vi "SeleccionarEntrada.vi"(6 "error in (no error)":errorcluster, 9 "DAQ in":refnum<class "DAQ.lvclass">) -> (0 "error out":errorcluster, 3 "DAQ out":refnum<class "DAQ.lvclass">)   [LabVIEW 2019, in "DAQ.lvclass"]
uses:
  DAQ.lvclass
  <resource>/objmgr/daqmx.rc
  <vilib>/DAQmx/create/channels.llb/DAQmx Create Channel (AI-Voltage-Basic).vi
  <vilib>/DAQmx/configure/timing.llb/DAQmx Timing (Sample Clock).vi
panel:
  out "SampClk.Rate":dbl
  in  "Number of Samples":i32=100
  in  "Sample Rate":dbl=1000.0
  in  "Sample Clock Source":tag="OnboardClock"
  in  "Terminal Configuration":i32(ring)=-1 items=["default"=-1, "RSE"=10083, "NRSE"=10078, "Differential"=10106, "Pseudodifferential"=12529]
  in  "Max Voltage":dbl=5.0
  in  "Min Voltage":dbl=-5.0
  in  "Physical Channel":tag="Dev1/ai0"
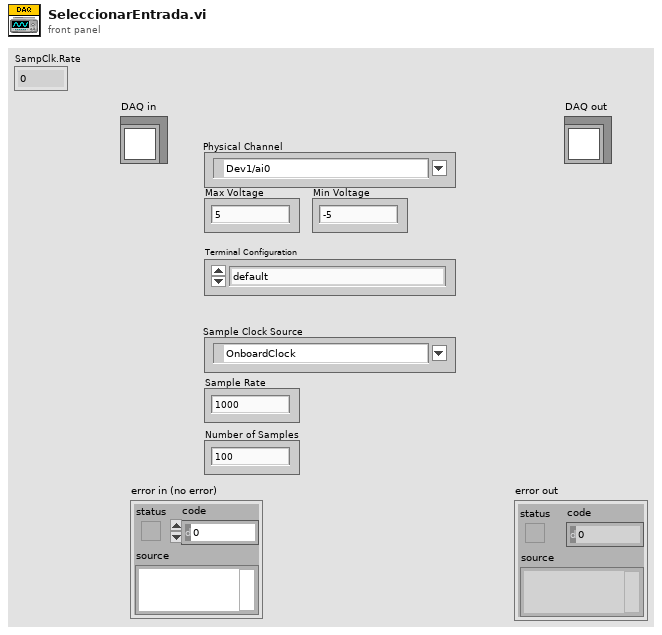
[diagram p1: front panel]
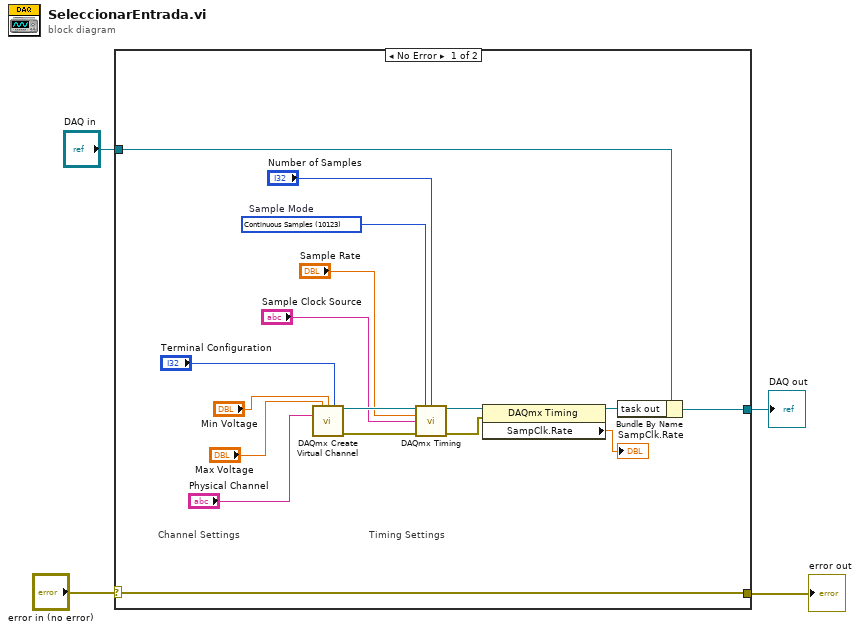
[diagram p0: block diagram]
diagram:
  n1 = case shown="No Error" "error in (no error)" {
    selector: "error in (no error)" -> [w15 w23]
    tunnel: [w15 w23] -> w4
    tunnel: [w5 w22] -> w1
    tunnel: "DAQ in" -> [w6 w22]
    frame No Error {
      w11 = 10123 items=["Finite Samples"=10178, "Continuous Samples"=10123, "Hardware Timed Single Point"=12522]  # Sample Mode
      # "Timing Settings"
      # "Channel Settings"
      n2 = call-poly <vilib>:"DAQmx Create Virtual Channel.vi"("maximum value"="Max Voltage", "minimum value"="Min Voltage", "input terminal configuration"="Terminal Configuration", "physical channels"="Physical Channel") -> ("task out"=w19:refnum<k21>, "error out"=w20:errorcluster)  [unwired: 10 in]
      n3 = call-poly <vilib>:"DAQmx Timing.vi"("task/channels in"=w19, "sample mode"=w11, "samples per channel"="Number of Samples", "rate"="Sample Rate", "source"="Sample Clock Source", "error in"=w20) -> ("task out"=w13:refnum<k21>, "error out"=w21:errorcluster)  [unwired: 8 in]
      n4 = property class="DAQmx Timing"(reference=w13, error in=w21) -> (reference out=w7:refnum<k21>, "SampClk.Rate"=→"SampClk.Rate":dbl)  [unwired: 1 out]
      n5 = Bundle By Name(cluster=w6, "task out"=w7) -> (w5:refnum<class "DAQ.lvclass">)
    }
    frame Error {
    }
  }
  "error out" <- w4
  "DAQ out" <- w1
